vi "Init.vi"(8 "error in":errorcluster, 10 "IConfigure":refnum<class "IConfigure.lvclass">, 11 "IRead Voltage in":refnum<class "IRead Voltage.lvclass">) -> (0 "error out":errorcluster, 3 "IRead Voltage out":refnum<class "IRead Voltage.lvclass">)   [LabVIEW 2023, in "HAL Interfaces.lvlib" / "IRead Voltage.lvclass"]
uses:
  IRead Voltage.lvclass
  IConfigure/IConfigure.lvclass
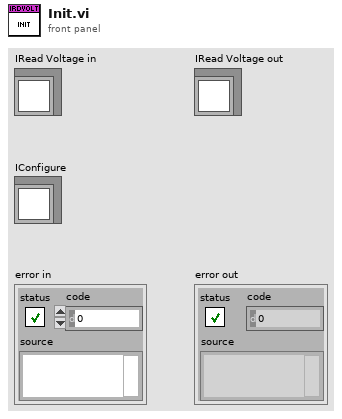
[diagram p1: front panel]
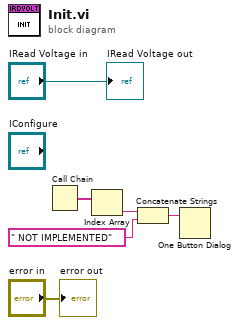
[diagram p0: block diagram]
diagram:
  n1 = Call Chain() -> (call chain=w4:string[])
  n2 = Index Array(array=w4) -> (element=w1:string)  [unwired: 1 in]
  n3 = Concatenate Strings(w1, " NOT IMPLEMENTED" ("string")) -> (w3:string)
  n4 = One Button Dialog(message=w3) -> ()  [unwired: 1 in, 1 out]
  "error out" <- "error in"
  "IRead Voltage out" <- "IRead Voltage in"
